vi "Boonoton_show_output_values.vi"() -> ()   [LabVIEW 2015]
uses:
  <vilib>/Instr/_visa.llb/GPIB Status Boolean Array.ctl
panel:
  out "External Bias [V]":dbl
  out "G [uS]":dbl
  out "Cp [pF]":dbl
  in  "Stop Button":bool
  out "data":string
  in  "mode (0)":i16
  out "ibsta":T1
  out "Error Out":errorcluster
  in  "Error In":errorcluster
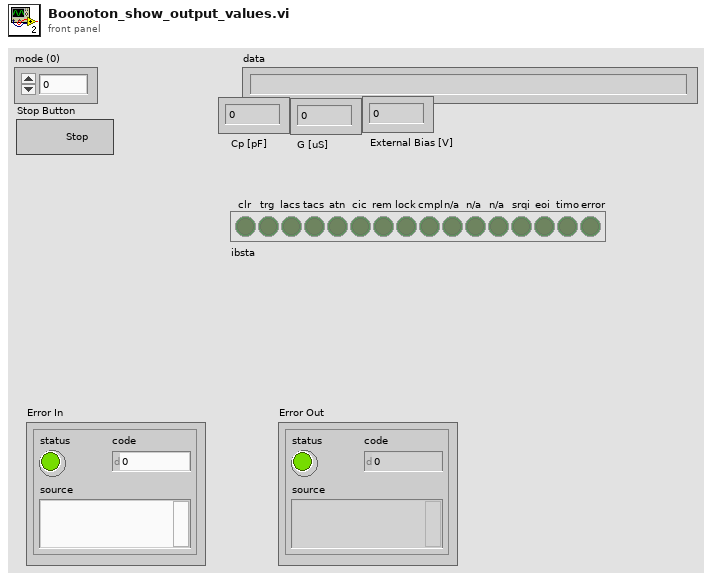
[diagram p1: front panel]
types:
  T1 = typedef "GPIB Status Boolean Array.ctl" = bool[]
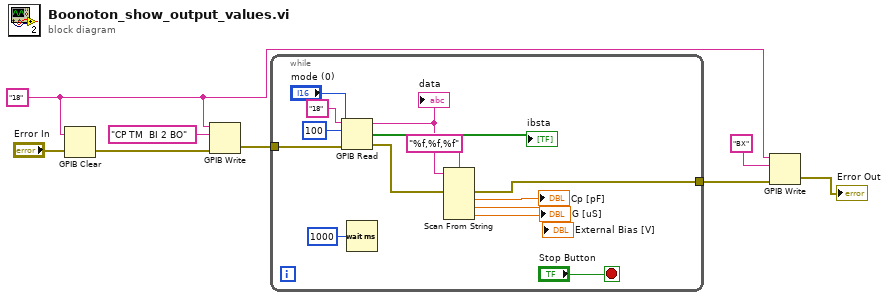
[diagram p0: block diagram]
diagram:
  w1 = "18"
  n1 = GPIB Clear(2:"Error In", 3:w1) -> (0:w8:errorcluster)  [unwired: 1 out]
  n2 = GPIB Write(0:w1, 1:"CP TM  BI 2 BO" ("data"), 3:w8) -> (6:w7:errorcluster)  [unwired: 2 in, 1 out]
  n3 = while {
    tunnel: w7 -> [w22]
    tunnel: [w14] -> w3
    stop <- "Stop Button" stop-if-true
    n4 = GPIB Read(0:"18" ("address string"), 1:100 ("byte count"), 2:"mode (0)", 3:w22) -> (5:w15:string, 6:→"ibsta":bool[], 7:w13:errorcluster)  [unwired: 1 in]
    "data" <- w15
    n5 = Wait (ms)(milliseconds to wait=u32 1000) -> ()  [unwired: 1 out]
    n6 = Scan From String(format string="%f,%f,%f", input string=w15, error in=w13) -> (error out=w14:errorcluster, output 1=→"Cp [pF]":dbl, output 2=→"G [uS]":dbl, output 3=→"External Bias [V]":dbl)  [unwired: 4 in, 2 out]
  }
  n7 = GPIB Write(0:w1, 1:"BX" ("data"), 3:w3) -> (6:→"Error Out":errorcluster)  [unwired: 2 in, 1 out]
